vi "Fetch and Save per partes.vi"(4 "variable prefix (data)":string="data", 5 "generate time axis (T)":bool, 6 "file format (mat)":T1(ring), 7 "channels":string[](array[string]), 8 "error in":errorcluster caption="error in (no error)", 10 "file path and name":path, 11 "instrument handles":refnum<k15>[](array[refnum])) -> (0 "error out":errorcluster, 1 "no of vars in matlab file":i32, 2 "sampling start times":timestamp[](array[timestamp]), 3 "instrument handles out":refnum<k15>[](array[refnum]))   [LabVIEW 2013, in "varilib.lvlib"]
doc: "Fetch all measured data from NI Scope type digitizers and save them to a file. It is done in parts thus vi is not limited by computer RAM and very large records can be transfered. File format is either a single text file with comma separated values or a Matlab binary holding multiple variables. These variables have to be concatenated in matlab/GNU Octave. A time axis can be generated. Returns value in how many times the process was repeated and a number of variables in binary format."
uses:
  varilib.lvlib
  <vilib>/Utility/error.llb/Error Cluster From Error Code.vi
  <instrlib>/niScope/Acquire/Fetch/niScope Multi Fetch WDT.vi
  <vilib>/Utility/file.llb/Write To Spreadsheet File (DBL).vi
  <vilib>/ErrorRing/Error Ring.xnode
panel:
  out "mat file renum":refnum<file>
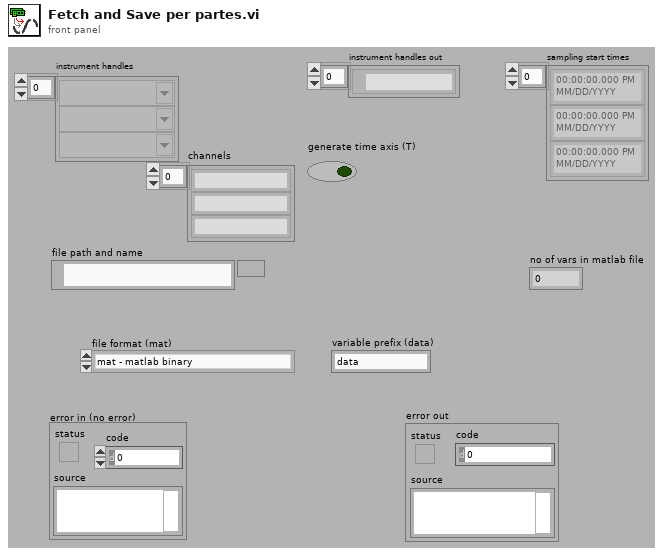
[diagram p1: front panel]
types:
  T1 = enum16{"mat - matlab binary", "csv - semicolon separated values"}
  T2 = enum16{"open", "replace", "create", "open or create", "replace or create", "replace or create with confirmation"}
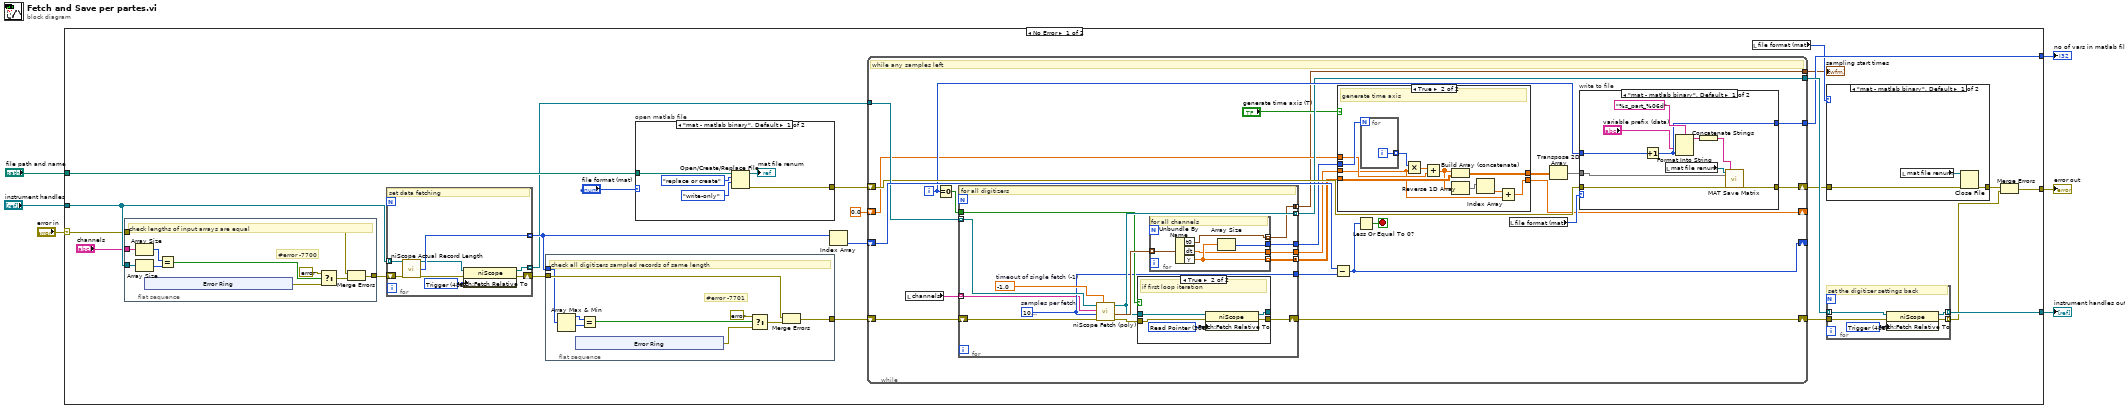
[diagram p0: block diagram]
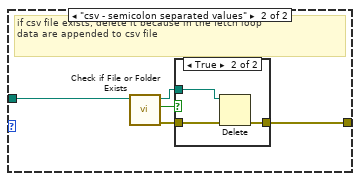
[diagram p3: hidden frame]
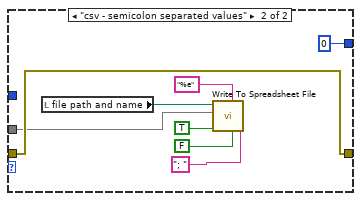
[diagram p7: hidden frame]
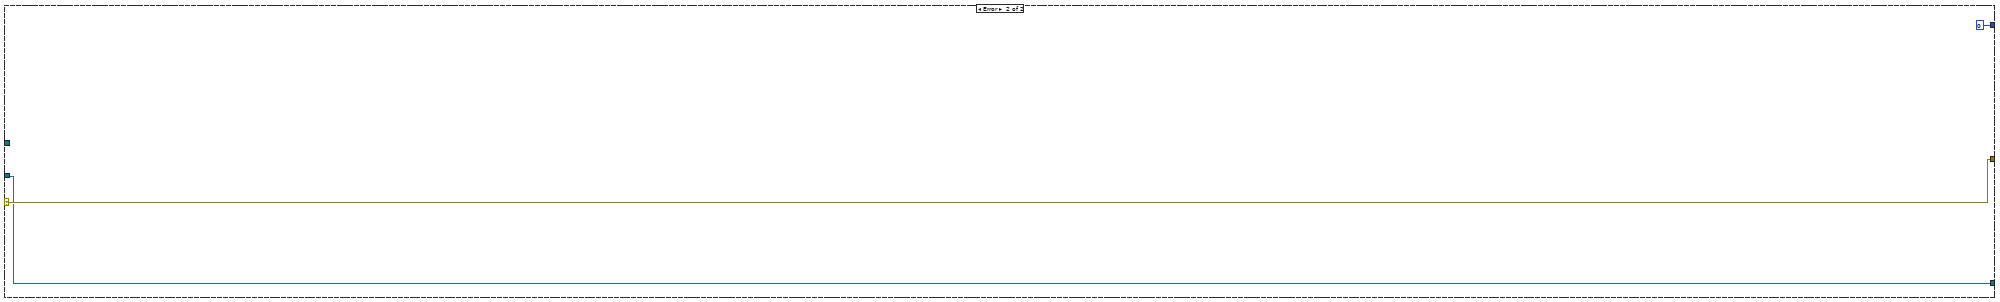
[diagram p8: hidden frame]
diagram:
  n1 = case shown="No Error" "error in" {
    selector: "error in" -> [w9 w174]
    tunnel: "instrument handles" -> [w11 w173]
    tunnel: [w27 w173] -> w1
    tunnel: [w23 w174] -> w5
    tunnel: "file path and name" -> [w21 _]
    tunnel: [w20 0] -> w3
    frame No Error {
      n2 = flat-sequence {
        tunnel: w11 -> [w53]
        tunnel: "channels" -> [w52]
        tunnel: w9 -> [w45]
        tunnel: [w44] -> w8
        frame #0 {
          # "#error -7700"
          # "check lengths of input arrays are equal"
          n3 = Array Size(array=w52) -> (size(s)=w47:i32)
          n4 = Array Size(array=w53) -> (size(s)=w48:i32)
          n5 = xnode "Error Ring"() -> ("error out"=w51:errorcluster)
          n6 = Equal?(x=w47, y=w48) -> (x = y?=w46:bool)
          n7 = Select(t=errorcluster {"status"=FALSE, "code"=0, "source"=""} ("f"), s=w46, f=w51) -> (s? t:f=w49:errorcluster)
          n8 = Merge Errors(w45, w49) -> (w44:errorcluster)
        }
      }
      n9 = for {
        tunnel: [w71] -> w16 mode=indexing
        tunnel: w11 -> [w70] mode=indexing
        tunnel: [w64] -> w12 mode=indexing
        shift-right: [w66] -> w17
        shift-left: w8 -> [w69]
        w68 = 483 items=["Start"=482, "Trigger"=483, "Pretrigger"=477, "Now"=481, "Read Pointer"=388] ("Fetch:Fetch Relative To")
        # "set data fetching"
        n10 = call <instrlib>:"niScope Actual Record Length.vi"("instrument handle"=w70, "error in"=w69) -> ("instrument handle out"=w65:refnum<k15>, "actual record length"=w71:i32, "error out"=w67:errorcluster)  [unwired: 11 in]
        n11 = property class="niScope"(reference=w65, error in=w67, "Fetch:Fetch Relative To"=w68) -> (reference out=w64:refnum<k15>, error out=w66:errorcluster)
      }
      n12 = flat-sequence {
        tunnel: w17 -> [w36]
        tunnel: w16 -> [w31]
        tunnel: [w30] -> w13
        frame #0 {
          # "#error -7701"
          # "check all digitizers sampled records of same length"
          n13 = Array Max & Min(array=w31) -> (max value=w38:i32, min value=w37:i32)  [unwired: 2 out]
          n14 = xnode "Error Ring"() -> ("error out"=w34:errorcluster)
          n15 = Equal?(x=w38, y=w37) -> (x = y?=w35:bool)
          n16 = Select(t=errorcluster {"status"=FALSE, "code"=0, "source"=""} ("f"), s=w35, f=w34) -> (s? t:f=w32:errorcluster)
          n17 = Merge Errors(w36, w32) -> (w30:errorcluster)
        }
      }
      n18 = case "open matlab file" shown="\"mat - matlab binary\", Default" "file format (mat)" {
        tunnel: w21 -> [w80 w85]
        tunnel: [w79 w82] -> w26
        frame "mat - matlab binary", Default {
          n19 = Open/Create/Replace File(file path (use dialog)=w80, operation (0:open)=T2."replace or create", access (0:read/write)=enum16{"read/write", "read-only", "write-only"}."write-only") -> (refnum out=→"mat file renum":refnum<file>, error out=w79:errorcluster)  [unwired: 3 in, 1 out]
        }
        frame "csv - semicolon separated values" {
          # "if csv file exists, delete it because in the fetch loop\ndata are appended to csv file"
          n20 = call <vilib>:"Check if File or Folder Exists.vi"("path"=w85) -> ("error out"=w83:errorcluster, "file or folder exists?"=w81:bool, "dup path"=w84:path)  [unwired: 8 in]
          n21 = case shown="True" w81 {
            tunnel: w84 -> [_ w89]
            tunnel: w83 -> [w86 w88]
            tunnel: [w86 w87] -> w82
            frame False {
            }
            frame True {
              n22 = Delete(path (use dialog)=w89, error in=w88) -> (error out=w87:errorcluster)  [unwired: 3 in, 2 out]
            }
          }
        }
      }
      n23 = Index Array(array=w16) -> (element=w15:i32)  [unwired: 1 in]
      n24 = while "While Loop per samples per fetch" {
        shift-right: [w111] -> _
        shift-left: w15 -> [w113]
        shift-right: [w102] -> w29
        shift-left: w13 -> [w110]
        shift-right: [w107] -> w25
        shift-left: w26 -> [w108]
        tunnel: [w105] -> w20
        tunnel: w12 -> [w109]
        tunnel: [w101] -> w28
        shift-right: [w95] -> _
        shift-left: 0.0 ("xIncrement") -> [w97]
        tunnel: [w90] -> w7
        i -> [w106]
        stop <- w112 stop-if-true
        # "while any samples left"
        n25 = local read "channels"() -> (w91:string[])
        n26 = Equal To 0?(x=w106) -> (x = 0?=w100:bool)
        n27 = for {
          tunnel: w109 -> [w140] mode=indexing
          tunnel: [w135] -> w101 mode=indexing
          tunnel: [w130] -> w103
          tunnel: [w137] -> w98 mode=concatenating
          shift-right: [w134] -> w102
          shift-left: w110 -> [w141]
          tunnel: w100 -> [w133]
          tunnel: [w132] -> w99
          tunnel: [w131] -> w96
          tunnel: w91 -> [w129] mode=indexing
          tunnel: [w128] -> w90 mode=concatenating
          w130 = 1000000  # samples per fetch
          w138 = -1.0  # timeout of single fetch (-1)
          # "for all digitizers"
          n28 = call-poly <instrlib>:"niScope Fetch (poly).vi"("timeout"=w138, "error in"=w141, "numSamples"=w130, "channels"=w129, "instrument handle"=w140) -> ("error out"=w136:errorcluster, "wfm"=w139:waveform(dbl)[], "instrument handle out"=w135:refnum<k15>)  [unwired: 3 in, 1 out]
          n29 = case shown="True" w133 {
            tunnel: w135 -> [w143 w148]
            tunnel: w136 -> [w142 w147]
            tunnel: [w143 w145] -> _
            tunnel: [w142 w144] -> w134
            frame False {
            }
            frame True {
              w146 = 388 items=["Start"=482, "Trigger"=483, "Pretrigger"=477, "Now"=481, "Read Pointer"=388] ("Fetch:Fetch Relative To")
              # "if first loop iteration"
              n30 = property class="niScope"(reference=w148, error in=w147, "Fetch:Fetch Relative To"=w146) -> (reference out=w145:refnum<k15>, error out=w144:errorcluster)
            }
          }
          n31 = for {
            tunnel: w139 -> [w152] mode=indexing
            tunnel: [w151] -> w137 mode=indexing
            tunnel: [w153] -> w132
            tunnel: [w150] -> w131
            tunnel: [w149] -> w128 mode=indexing
            # "for all channels"
            n32 = Unbundle By Name(w152) -> ("t0"=w149:timestamp, "dt"=w150:dbl, "Y"=w151:dbl[])
            n33 = Array Size(array=w151) -> (size(s)=w153:i32)
          }
        }
        n34 = Subtract(x=w113, y=w103) -> (x-y=w111:i32)
        n35 = case shown="True" "generate time axis (T)" {
          tunnel: [w115 w116] -> w93
          tunnel: w99 -> [_ w126]
          tunnel: w98 -> [w115 w125]
          tunnel: w97 -> [_ w124]
          tunnel: w96 -> [w114 w123]
          tunnel: [w114 w122] -> w95
          frame False {
          }
          frame True {
            # "generate time axis"
            n36 = for {
              N: w126 -> [_]
              tunnel: [w127] -> w121 mode=indexing
              i -> [w127]
            }
            n37 = Multiply(x=w121, y=w123) -> (x*y=w120:dbl[])
            n38 = Add(x=w120, y=w124) -> (x+y=w119:dbl[])
            n39 = Build Array (concatenate)(w119, w125) -> (w116:dbl[][])
            n40 = Reverse 1D Array(array=w119) -> (reversed array=w118:dbl[])
            n41 = Index Array(array=w118) -> (element=w117:dbl)  [unwired: 1 in]
            n42 = Add(x=w117, y=w123) -> (x+y=w122:dbl)
          }
        }
        n43 = Less Or Equal To 0?(x=w111) -> (x <= 0?=w112:bool)
        n44 = local read "file format (mat)"() -> (w104:T1)
        n45 = Transpose 2D Array(2D array=w93) -> (transposed array=w92:dbl[][])
        n46 = case "write to file" shown="\"mat - matlab binary\", Default" w104 {
          tunnel: w92 -> [w163 w164]
          tunnel: w108 -> [w162 w167]
          tunnel: [w161 w167] -> w107
          tunnel: w106 -> [w157 _]
          tunnel: [w156 0] -> w105
          frame "mat - matlab binary", Default {
            n47 = Increment(x=w157) -> (x+1=w156:i32)
            n48 = local read "mat file renum"() -> (w154:refnum<file>)
            n49 = Format Into String(format string="%s_part_%06d", "variable prefix (data)", w156) -> (resulting string=w158:string)  [unwired: 2 in, 1 out]
            n50 = Concatenate Strings(w158) -> (w160:string)
            n51 = call "MAT Save Matrix.vi"("Ref Num"=w154, "DBL"=w163, "error in"=w162, "Matrix Name"=w160) -> ("error out"=w161:errorcluster)  [unwired: 14 in, 1 out]
          }
          frame "csv - semicolon separated values" {
            n52 = local read "file path and name"() -> (w165:path)
            n53 = call-poly <vilib>:"Write To Spreadsheet File.vi"("delimiter (\\t)"="; " ("delimiter (\\t)"), "transpose? (no:F)"=FALSE, "format (%.3f)"="%e" ("format (%d)"), "append to file? (new file:F)"=TRUE, "2D data"=w164, "file path (dialog if empty)"=w165) -> ()  [unwired: 2 in, 1 out]
          }
        }
      }
      "sampling start times" <- w7
      n54 = local read "file format (mat)"() -> (w19:T1)
      n55 = case shown="\"mat - matlab binary\", Default" w19 {
        tunnel: w25 -> [w74 w75]
        tunnel: [w73 w75] -> w22
        frame "mat - matlab binary", Default {
          n56 = local read "mat file renum"() -> (w72:refnum<file>)
          n57 = Close File(refnum=w72, error in=w74) -> (error out=w73:errorcluster)  [unwired: 1 out]
        }
        frame "csv - semicolon separated values" {
        }
      }
      n58 = for {
        tunnel: w29 -> [w63]
        tunnel: w28 -> [w62] mode=indexing
        tunnel: [w61] -> w27 mode=indexing
        tunnel: [w60] -> w24 mode=indexing
        w59 = 483 items=["Start"=482, "Trigger"=483, "Pretrigger"=477, "Now"=481, "Read Pointer"=388] ("Fetch:Fetch Relative To")
        # "set the digitizer settings back"
        n59 = property class="niScope"(reference=w62, error in=w63, "Fetch:Fetch Relative To"=w59) -> (reference out=w61:refnum<k15>, error out=w60:errorcluster)
      }
      n60 = Merge Errors(w22, w24) -> (w23:errorcluster)
    }
    frame Error {
    }
  }
  "error out" <- w5
  "no of vars in matlab file" <- w3
  "instrument handles out" <- w1
